vi "NewProjectNameDialog.vi"() -> (1 "Project Name Out":string, 3 "Cancel?":bool)   [LabVIEW 2014, in "Project.lvclass"]
uses:
  Project.lvclass
panel:
  in  "Project Name":string
  in  "Cancel":bool
  in  "OK":bool
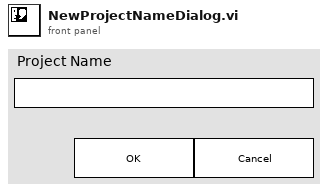
[diagram p1: front panel]
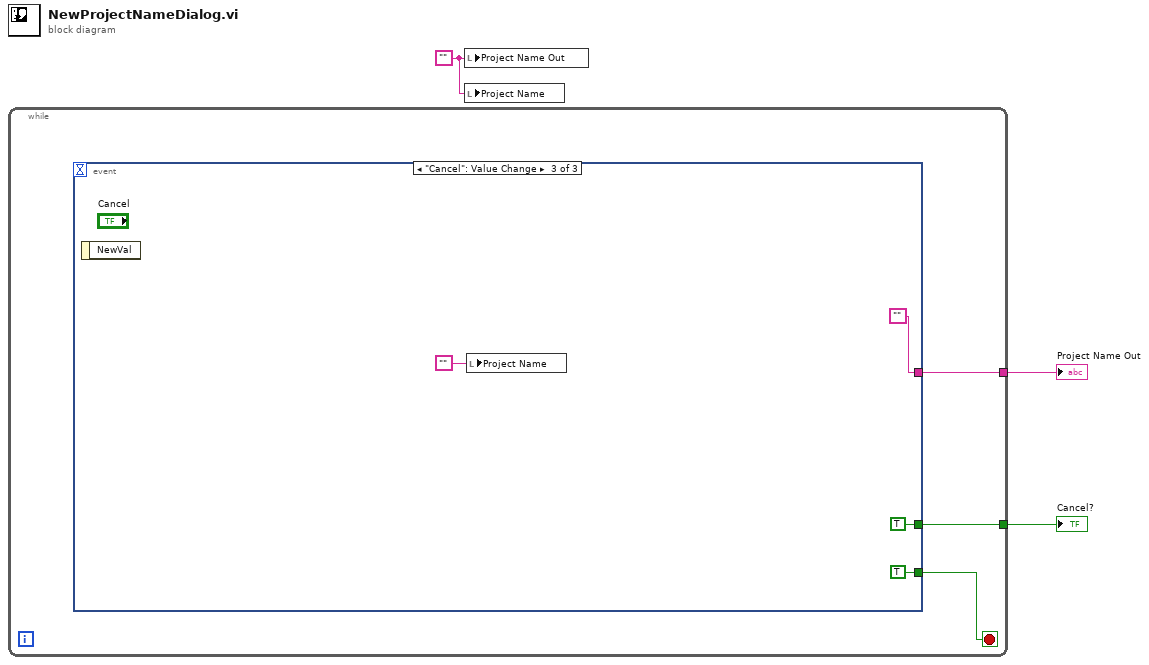
[diagram p0: block diagram]
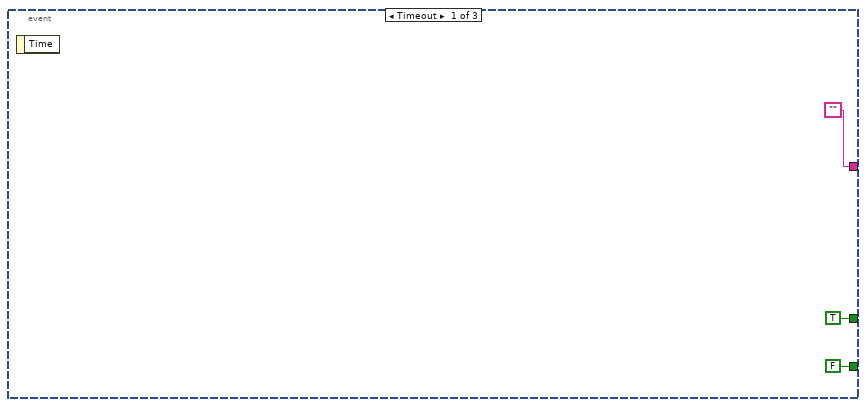
[diagram p2: hidden frame]
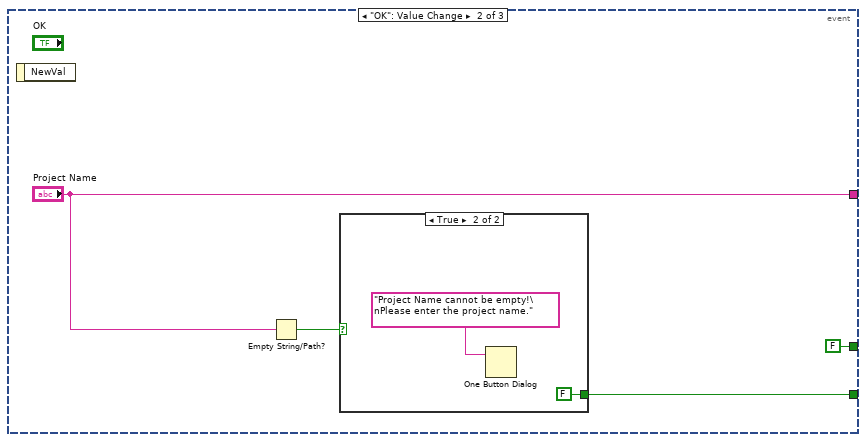
[diagram p3: hidden frame]
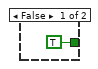
[diagram p4: hidden frame]
diagram:
  w1 = "" ("Step Name Out")
  n1 = while {
    tunnel: [w5] -> w3
    tunnel: [w4] -> w2
    stop <- w6 stop-if-true
    n2 = event shown="[2] \"Cancel\": Value Change" {
      selector: _ -> [_ _ _]
      dyn-events: _ -> [_ _ _]
      timeout: _ -> [_ _ _]
      tunnel: [FALSE w10 TRUE] -> w6
      tunnel: [TRUE FALSE TRUE] -> w5
      tunnel: ["" ("Step Name") "Project Name" "" ("Step Name")] -> w4
      event Timeout {
        n3 = event-data() -> ()  [unwired: 1 in, 1 out]
      }
      event "OK": Value Change {
        n4 = event-data() -> ()  [unwired: 1 in, 1 out]
        n5 = Empty String/Path?(string/path="Project Name") -> (empty?=w12:bool)
        n6 = case shown="True" w12 {
          tunnel: [TRUE FALSE] -> w10
          frame False {
          }
          frame True {
            n7 = One Button Dialog(message="Project Name cannot be empty!\nPlease enter the project name.") -> ()  [unwired: 1 in, 1 out]
          }
        }
      }
      event "Cancel": Value Change {
        n8 = event-data() -> ()  [unwired: 1 in, 1 out]
        n9 = local write "Project Name"("" ("Step Name Out")) -> ()
      }
    }
  }
  "Cancel?" <- w3
  "Project Name Out" <- w2
  n10 = local write "Project Name Out"(w1) -> ()
  n11 = local write "Project Name"(w1) -> ()
